vi "ProdaNG.Tree.Release.vi"(6 "comment":string, 7 "TestStepsTree":refnum<vi>, 8 "error in (no error)":errorcluster, 9 "Release":bool, 10 "Elements to release/unrelease":T1[](array[typedef]), 11 "dbHandleIn":i32) -> (0 "error out":errorcluster, 3 "dbHandle":i32)   [LabVIEW 2016]
uses:
  ProdaNG.Tree.Fglb.Data.ctl
  ProdaNG.Tree.Fglb.Element.ctl
  Controls/ProdaNG.ReleaseId.ctl
  ProdaNG.Configurator.Glb.vi
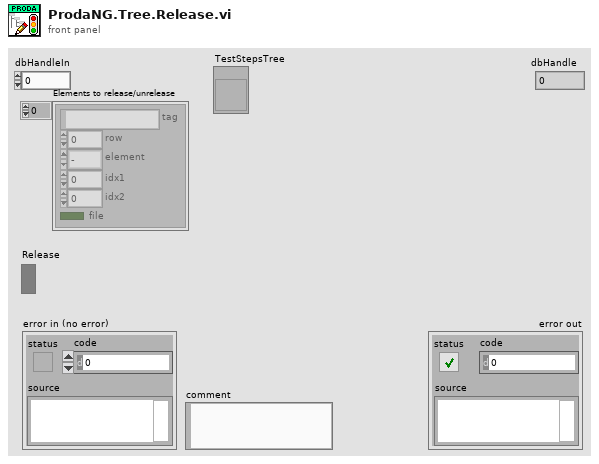
[diagram p1: front panel]
types:
  T1 = typedef "ProdaNG.Tree.Fglb.Data.ctl" = cluster{"tag":string, "row":i32, "element":T2, "idx1":i32, "idx2":i32, "file":bool}
  T2 = typedef "ProdaNG.Tree.Fglb.Element.ctl" = enum16{"-", "PP", "TS", "TP", "TV"}
  T3 = typedef "ProdaNG.ReleaseId.ctl" = enum16{"not released", "released", "was released"}
  T4 = typedef "ProdaNG.TestStep.ctl" = cluster{"i_id":i32, "processStepId":i32, "testSequence":i32, "testOrder":i32, "mdReason":string, "mdUser":string, "mdTime":string, "description":string}
  T5 = typedef "ProdaNG.TestStepParam.ctl" = cluster{"i_id":i32, "testStepId":i32, "unitId":i32, "contentId":string, "previewId":string, "value":dbl, "valueText":string, "paramSequence":i32, "history":i32, "mdReason":string, "mdUser":string, "mdTime":string, "description":string}
  T6 = typedef "ProdaNG.TestValue.ctl" = cluster{"i_id":i32, "testStepId":i32, "releaseId":i32, "unitId":i32, "contentId":string, "previewId":string, "maximum":dbl, "minimum":dbl, "valueText":string, "testValueSequence":i32, "history":i32, "mdReason":string, "mdUser":string, "mdTime":string, "description":string}
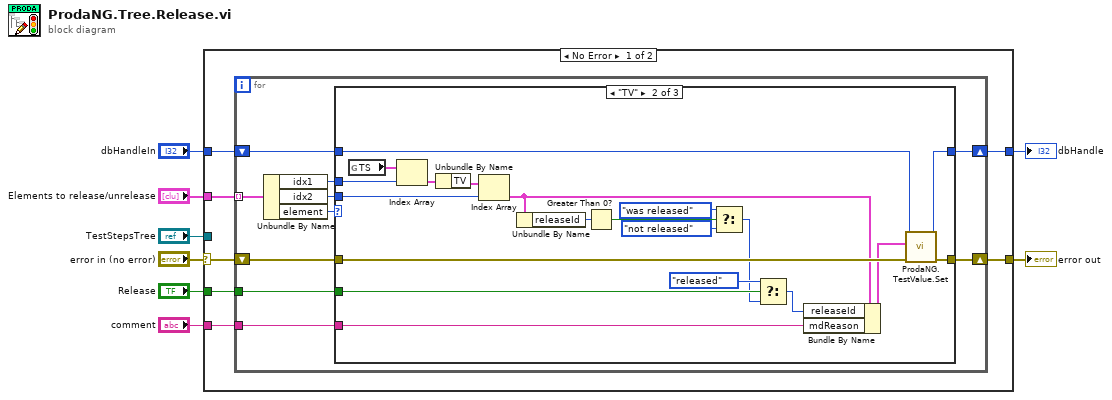
[diagram p0: block diagram]
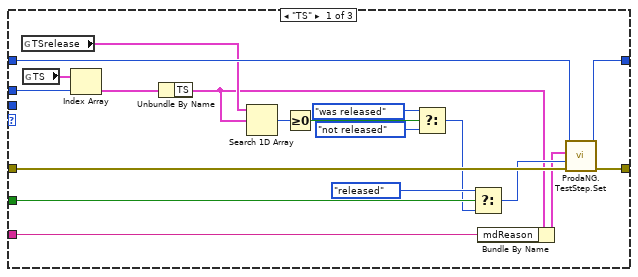
[diagram p2: hidden frame]
diagram:
  n1 = case shown="No Error" "error in (no error)" {
    selector: "error in (no error)" -> [w9 w68]
    tunnel: "TestStepsTree" -> [_ _]
    tunnel: [w15 w68] -> w8
    tunnel: "dbHandleIn" -> [w14 w67]
    tunnel: [w13 w67] -> w4
    tunnel: "Release" -> [w12 _]
    tunnel: "comment" -> [w11 _]
    tunnel: "Elements to release/unrelease" -> [w10 _]
    frame No Error {
      n2 = for {
        shift-right: [w23] -> w15
        shift-left: w9 -> [w17]
        shift-right: [w21] -> w13
        shift-left: w14 -> [w22]
        tunnel: w12 -> [w20]
        tunnel: w11 -> [w19]
        tunnel: w10 -> [w18] mode=indexing
        n3 = Unbundle By Name(w18) -> ("idx1"=w24:i32, "idx2"=w16:i32, "element"=w25:T2)
        n4 = case shown="\"TV\"" w25 {
          tunnel: w24 -> [w44 w64 _]
          tunnel: w17 -> [w42 w62 w66]
          tunnel: [w41 w61 w66] -> w23
          tunnel: w22 -> [w40 w60 w65]
          tunnel: [w39 w59 w65] -> w21
          tunnel: w20 -> [w37 w56 _]
          tunnel: w19 -> [w38 w58 _]
          tunnel: w16 -> [_ w48 _]
          frame "TS" {
            n5 = global read "ProdaNG.Configurator.Glb.vi" "TSrelease"() -> (w32:T4[])
            n6 = global read "ProdaNG.Configurator.Glb.vi" "TS"() -> (w43:cluster{"TS":T4, "TP":T5[], "TV":T6[]}[])
            n7 = Index Array(array=w43, index=w44) -> (element=w31:cluster{"TS":T4, "TP":T5[], "TV":T6[]})
            n8 = Unbundle By Name(w31) -> ("TS"=w26:T4)
            n9 = Search 1D Array(1D array=w32, element=w26) -> (index of element=w29:i32)  [unwired: 1 in]
            n10 = Greater Or Equal To 0?(x=w29) -> (x >= 0?=w28:bool)
            n11 = Select(t=ProdaNG.ReleaseId."was released" ("ReleaseId"), s=w28, f=ProdaNG.ReleaseId."not released" ("ReleaseId")) -> (s? t:f=w27:T3)
            n12 = Select(t=ProdaNG.ReleaseId."released" ("ReleaseId"), s=w37, f=w27) -> (s? t:f=w33:T3)
            n13 = Bundle By Name(cluster=w26, "mdReason"=w38) -> (w30:T4)
            n14 = call "ProdaNG.TestStep.Set.vi"("error in (no error)"=w42, "ReleaseId"=w33, "TestStep"=w30, "dbHandleIn"=w40) -> ("error out"=w41:errorcluster, "dbHandle"=w39:i32)  [unwired: 5 in, 1 out]
          }
          frame "TV" {
            n15 = global read "ProdaNG.Configurator.Glb.vi" "TS"() -> (w63:cluster{"TS":T4, "TP":T5[], "TV":T6[]}[])
            n16 = Index Array(array=w63, index=w64) -> (element=w49:cluster{"TS":T4, "TP":T5[], "TV":T6[]})
            n17 = Unbundle By Name(w49) -> ("TV"=w47:T6[])
            n18 = Index Array(array=w47, index=w48) -> (element=w46:T6)
            n19 = Unbundle By Name(w46) -> ("releaseId"=w50:i32)
            n20 = Greater Than 0?(x=w50) -> (x > 0?=w55:bool)
            n21 = Select(t=ProdaNG.ReleaseId."was released" ("ReleaseId"), s=w55, f=ProdaNG.ReleaseId."not released" ("ReleaseId")) -> (s? t:f=w51:T3)
            n22 = Select(t=ProdaNG.ReleaseId."released" ("ReleaseId"), s=w56, f=w51) -> (s? t:f=w45:T3)
            n23 = Bundle By Name(cluster=w46, "releaseId"=w45, "mdReason"=w58) -> (w57:T6)
            n24 = call "ProdaNG.TestValue.Set.vi"("error in (no error)"=w62, "TestValue"=w57, "dbHandleIn"=w60) -> ("error out"=w61:errorcluster, "dbHandle"=w59:i32)  [unwired: 6 in, 1 out]
          }
          frame Default {
          }
        }
      }
    }
    frame Error {
    }
  }
  "error out" <- w8
  "dbHandle" <- w4
